vi "SCPI_popout_write_read.vi"(8 "error in (no error)":errorcluster, 11 "VISA":refnum<visa-resource-name>) -> (0 "error out":errorcluster, 3 "VISA resource name out":refnum<visa-resource-name>)   [LabVIEW 2020]
uses:
  controls/SCPI_enum.ctl
panel:
  in  "GO":bool
  in  "stop":bool
  out "read numeric value":dbl
  out "read buffer - string":string
  in  "Numeric entrece":dbl
  in  "SCIPI":T1 items=["*IDN?", "*SAV 1", "*RCL 1", "INSTTrument CH1", "INSTTrument CH2", "INSTrument?", "MEASure:CURRent? CH1", "MEASure:CURRent? CH2", "MEASure:VOLTage? CH1", "MEASure:VOLTage? CH2", "MEASure:POWEr? CH1", "MEASure:POWEr? CH2", "CH1:CURRent?", "CH2:CURRent?", "CH1:VOLTage? ", "CH2:VOLTage? ", "OUTPut CH1,ON", "OUTPut CH1,OFF", "OUTPut CH2,ON", "OUTPut CH2,OFF", "OUTPut CH3,ON", "OUTPut CH3,OFF", "OUTPut:TRACK 0", "OUTPut:TRACK 1", "OUTPut:TRACK 2", "OUTPut:WAVE CH1,ON", "OUTPut:WAVE CH1,OFF", "OUTPut:WAVE CH2,ON", "OUTPut:WAVE CH2,OFF"]
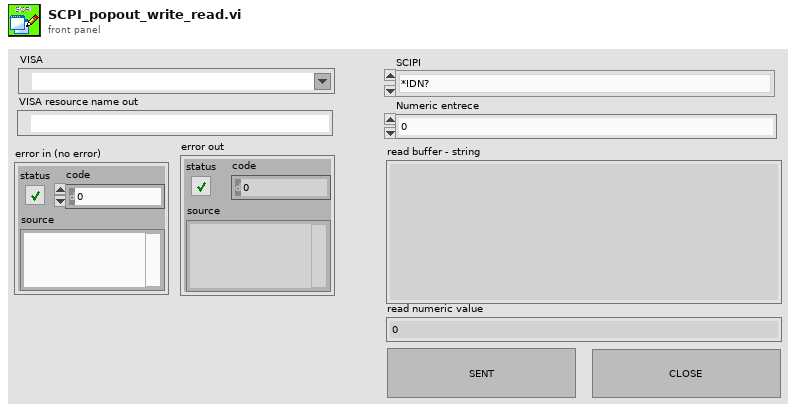
[diagram p1: front panel]
types:
  T1 = typedef "SCPI_enum.ctl" = u16
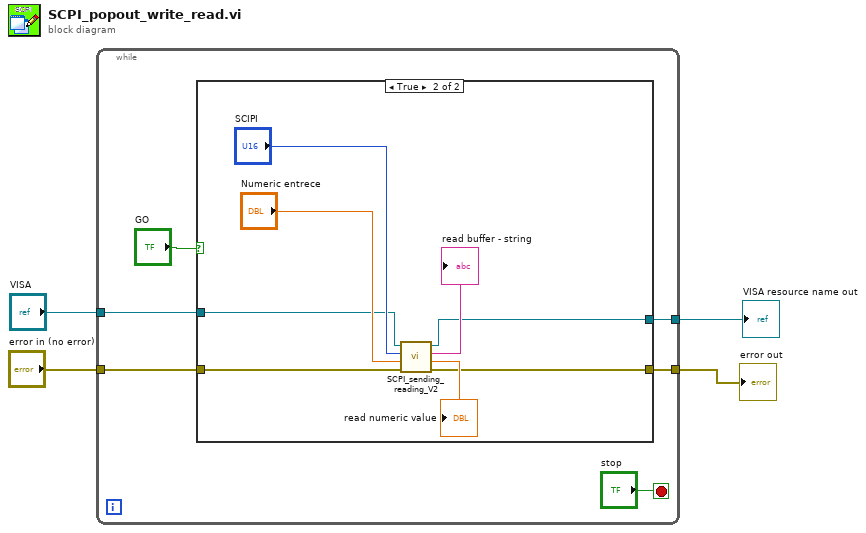
[diagram p0: block diagram]
diagram:
  n1 = while {
    tunnel: [w8] -> w4
    tunnel: [w7] -> w3
    tunnel: "VISA" -> [w6]
    tunnel: "error in (no error)" -> [w5]
    stop <- "stop" stop-if-true
    n2 = case shown="True" "GO" {
      tunnel: [w11 w16] -> w8
      tunnel: [w12 w15] -> w7
      tunnel: w6 -> [w12 w14]
      tunnel: w5 -> [w11 w13]
      frame False {
      }
      frame True {
        n3 = call "SCPI_sending_reading_V2.vi"("error in (no error)"=w13, "Numeric entrece"="Numeric entrece", "SCIPI"="SCIPI", "VISA"=w14) -> ("error out"=w16:errorcluster, "read numeric value"=→"read numeric value":dbl, "read buffer - string"=→"read buffer - string":string, "VISA resource name out"=w15:refnum<visa-resource-name>)
      }
    }
  }
  "error out" <- w4
  "VISA resource name out" <- w3
